vi "PSAE_VCH_Command.vi"(8 "Error In (no error)":errorcluster, 10 "Data":variant, 11 "Comd":T1(ring)) -> (0 "Error Out":errorcluster)   [LabVIEW 2016]
panel:
  # "Data Out"
  # "Data In"
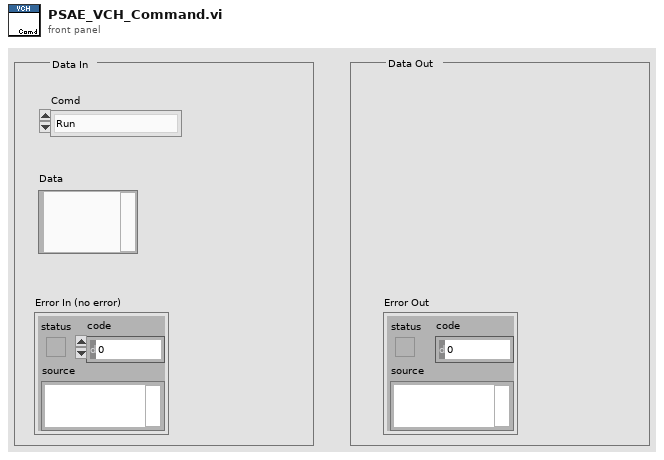
[diagram p1: front panel]
types:
  T1 = enum16{"Run", "Pause", "Stop", "DAQ Chl", "Save", "Update Data", "Symbol Path", "DAQ DATA Queues", "None"}
  T2 = cluster{"Main Queue":string, "DAQ Queue":string, "ANA Queue":string, "CUI Queue":string, "DRP Queue":string, "Graph Queue":string, "DOM Queue":string, "ACQ Queue":string, "MOD Queue":string, "OAA Queue":string, "REG Queue":string, "DRV Queue":string, "GEF Queue":string, "OVV Queue":string}
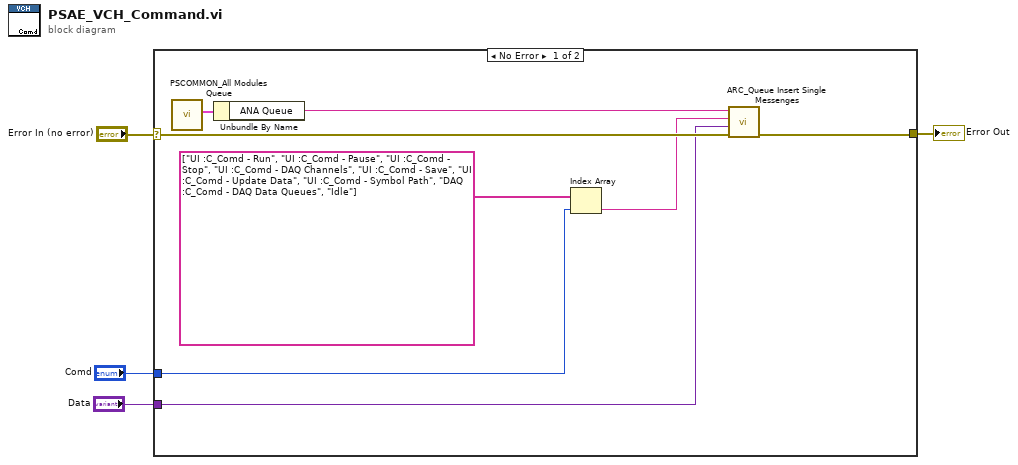
[diagram p0: block diagram]
diagram:
  n1 = case shown="No Error" "Error In (no error)" {
    selector: "Error In (no error)" -> [w12 w13]
    tunnel: [w11 w13] -> w4
    tunnel: "Comd" -> [w9 _]
    tunnel: "Data" -> [w7 _]
    frame No Error {
      n2 = call "PSCOMMON_All Modules Queue.vi"() -> ("All Queues"=w6:T2)  [unwired: 11 in]
      n3 = Unbundle By Name(w6) -> ("ANA Queue"=w5:string)
      n4 = Index Array(array=string[] ["UI :C_Comd - Run", "UI :C_Comd - Pause", "UI :C_Comd - Stop", "UI :C_Comd - DAQ Channels", "UI :C_Comd - Save", "UI :C_Comd - Update Data", "UI :C_Comd - Symbol Path", "DAQ :C_Comd - DAQ Data Queues", "Idle"], index=w9) -> (element=w8:string)
      n5 = call "ARC_Queue Insert Single Messenges.vi"("error in (no error)"=w12, "Data"=w7, "Order"=w8, "Queue Name"=w5) -> ("error out"=w11:errorcluster)  [unwired: 7 in]
    }
    frame Error {
    }
  }
  "Error Out" <- w4
